vi "CANFD Set Relay.vi"(8 "error in (no error)":errorcluster, 10 "RelayState":u8, 11 "DevHandle":i32) -> (0 "error out":errorcluster, 3 "function return":i32)   [LabVIEW 2010, in "usb2canfd.lvlib"]
doc: "int WINAPI CANFD_SetRelay(int DevHandle, unsigned char RelayState);"
uses:
  usb2canfd.lvlib
  USB2XXX/trunk/USB2XXX/USB2XXX/vs2010/Release/USB2XXX.dll
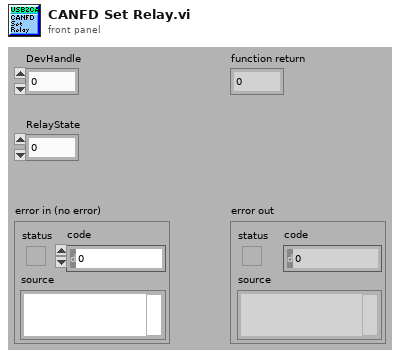
[diagram p1: front panel]
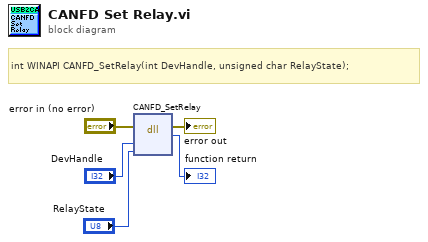
[diagram p0: block diagram]
diagram:
  # "int WINAPI CANFD_SetRelay(int DevHandle, unsigned char RelayState);"
  n1 = dll-call lib="E:/OtherWork/STM32/USB2XXX/trunk/USB2XXX/USB2XXX/vs2010/Release/USB2XXX.*" fn="CANFD_SetRelay"(error in="error in (no error)", "DevHandle"="DevHandle", "RelayState"="RelayState") -> (error out=→"error out":errorcluster, →"function return":i32)  [unwired: 4 in, 1 out]
